vi "Factorial.vi"() -> ()   [LabVIEW 2019]
panel:
  in  "Numeric 3":i32=1
  out "Numeric 2":i32
  in  "Numeric":u8
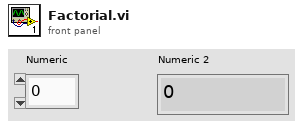
[diagram p1: front panel]
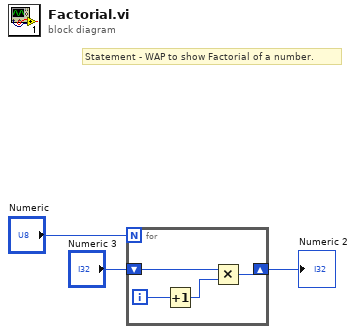
[diagram p0: block diagram]
diagram:
  # "Statement - WAP to show Factorial of a number."
  n1 = for {
    N: "Numeric" -> [_]
    shift-right: [w6] -> w3
    shift-left: "Numeric 3" -> [w7]
    i -> [w5]
    n2 = Increment(x=w5) -> (x+1=w4:i32)
    n3 = Multiply(x=w7, y=w4) -> (x*y=w6:i32)
  }
  "Numeric 2" <- w3
